vi "Emergency Stop.vi"(8 "error in":errorcluster, 11 "Light Stack in":refnum<class "Light Stack.lvclass">) -> (0 "error out":errorcluster, 3 "Light Stack out":refnum<class "Light Stack.lvclass">)   [LabVIEW 2018, in "Light Stack.lvlib" / "Light Stack.lvclass"]
uses:
  Light Stack.lvclass
  Custom Controls/Light Select.ctl
  Custom Controls/Light Mode.ctl
  Light Stack.lvlib
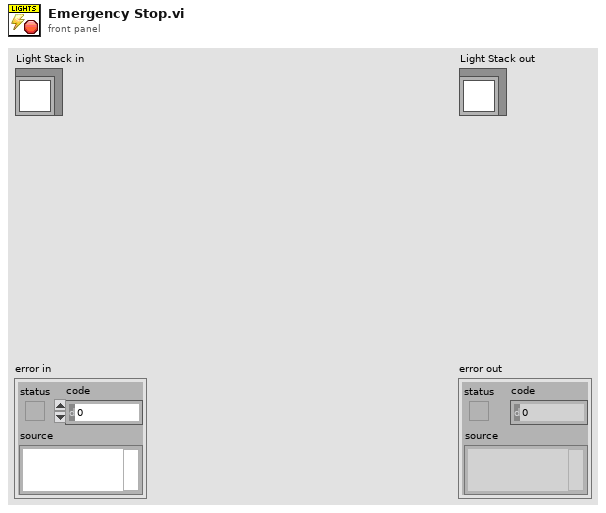
[diagram p1: front panel]
types:
  T1 = typedef "Light Stack.lvlib/Light Mode.ctl" = enum16{"OFF", "ON", "BLINK"}
  T2 = typedef "Light Stack.lvlib/Light Select.ctl" = enum16{"Red", "Amber", "Green", "Blue"}
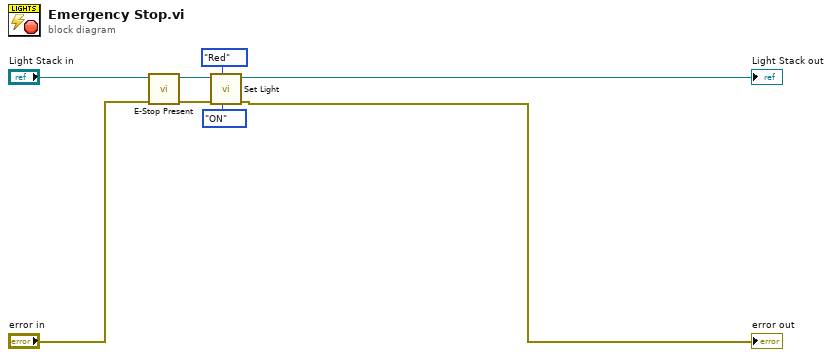
[diagram p0: block diagram]
diagram:
  n1 = call "E-Stop Present.vi"("error in"="error in", "Light Stack in"="Light Stack in") -> ("error out"=w6:errorcluster, "Light Stack out"=w5:refnum<class "Light Stack.lvclass">)  [unwired: 8 in]
  n2 = call "Set Light.vi"("State"=Light_Mode."ON", "Light Select"=Light_Select."Red", "error in"=w6, "Light Stack in"=w5) -> ("error out"=→"error out":errorcluster, "Light Stack out"=→"Light Stack out":refnum<class "Light Stack.lvclass">)  [unwired: 6 in]
